vi "Pick Image.vi"(5 "Image to Add [ ]":T1, 9 "String":string, 11 "error in (no error)":errorcluster) -> (4 "InstanceImage":refnum<k24>, 6 "Valid Image?":bool, 8 "String OUT":string, 10 "Change Font Color?":bool, 15 "error out":errorcluster)   [LabVIEW 2012]
doc: "Version 1.0\nDeveloped by Jean-Marc Simard\nCopyright © 2010, Exaprom Inc.\nAll rights reserved.\nLicense: BSD\n\nWith iTextSharp 4.1.6 (http://itextsharp.sourceforge.net)\nunder Mozilla Public License Version 1.1\n(http://www.mozilla.org/MPL/MPL-1.1.html)"
uses:
  Controls/Image to Add refnum [ ].ctl
  C:/Users/MaxCorp/Documents/TopPerm - Base/DLL/itextsharp.dll
  DLL/itextsharp.dll
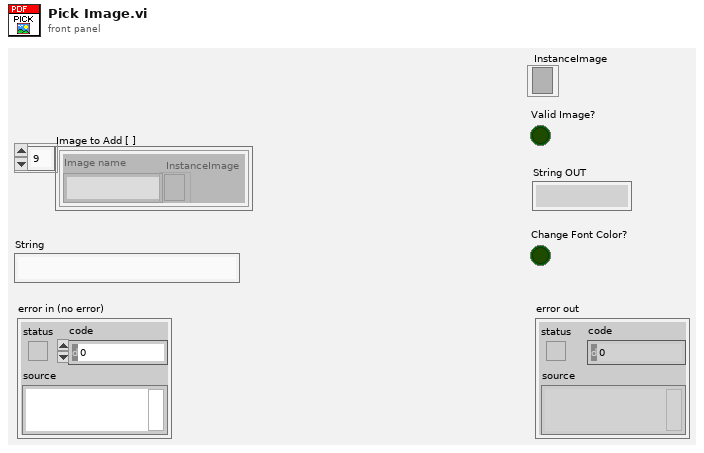
[diagram p1: front panel]
types:
  T1 = typedef "Image to Add refnum [ ].ctl" = cluster{"Image name":string, "InstanceImage":refnum<k24>}[]
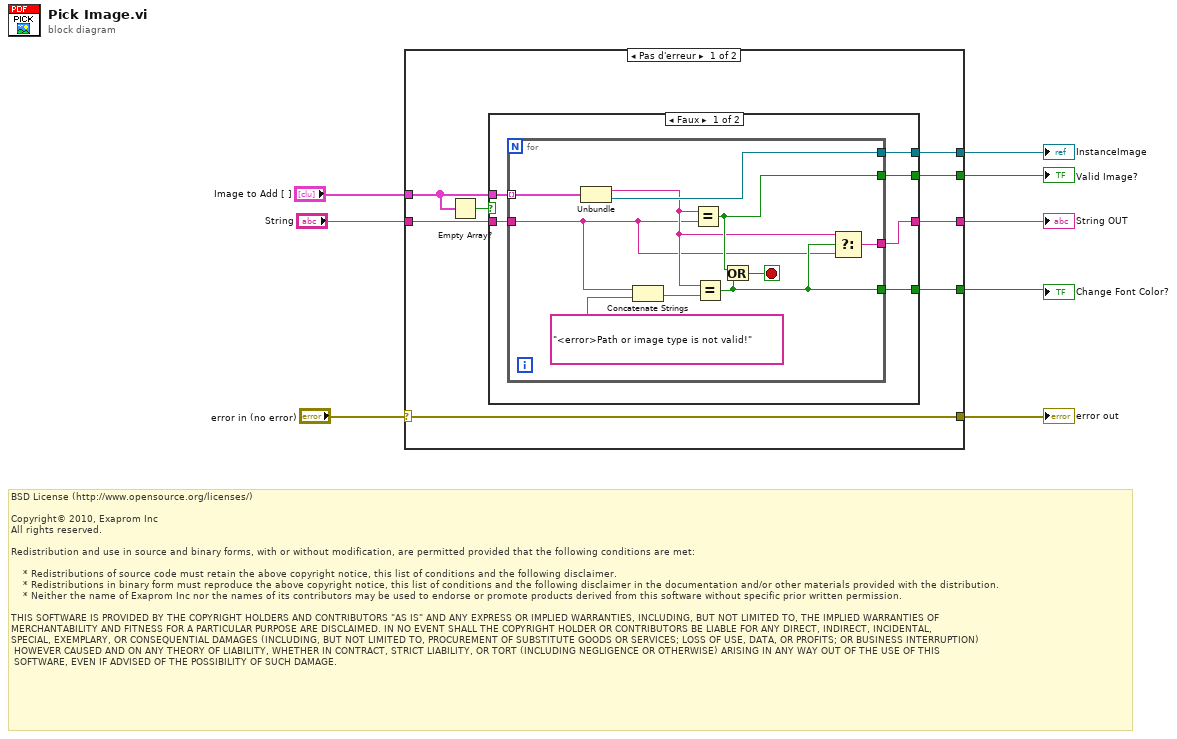
[diagram p0: block diagram]
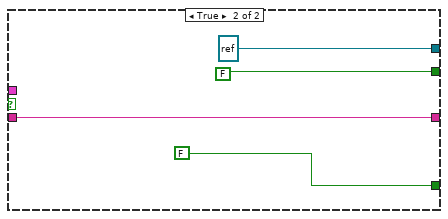
[diagram p2: hidden frame]
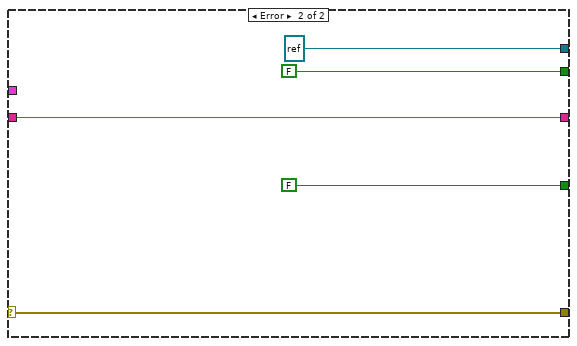
[diagram p3: hidden frame]
diagram:
  # "BSD License (http://www.opensource.org/licenses/)\n\nCopyright© 2010, Exaprom Inc\nAll rights reserved.\n\nRedistribution and use in source and binary forms, with or without modification, are permitted provided that the following conditions are met:\n\n    * Redistributions of source code must retain the above copyright notice, this list of conditions and the following disclaimer.\n    * Redistributions in binary form must reproduce the above copyright notice, this list of conditions and the following disclaimer in the documentation and/or other materials provided with the distribution.\n    * Neither the name of Exaprom Inc nor the names of its contributors may be used to endorse or promote products derived from this software without specific prior written permission.\n\nTHIS SOFTWARE IS PROVIDED BY THE COPYRIGHT HOLDERS AND CONTRIBUTORS \"AS IS\" AND ANY EXPRESS OR IMPLIED WARRANTIES, INCLUDING, BUT NOT LIMITED TO, THE IMPLIED WARRANTIES OF \nMERCHANTABILITY AND FITNESS FOR A PARTICULAR PURPOSE ARE DISCLAIMED. IN NO EVENT SHALL THE COPYRIGHT HOLDER OR CONTRIBUTORS BE LIABLE FOR ANY DIRECT, INDIRECT, INCIDENTAL,\nSPECIAL, EXEMPLARY, OR CONSEQUENTIAL DAMAGES (INCLUDING, BUT NOT LIMITED TO, PROCUREMENT OF SUBSTITUTE GOODS OR SERVICES; LOSS OF USE, DATA, OR PROFITS; OR BUSINESS INTERRUPTION)\n HOWEVER CAUSED AND ON ANY THEORY OF LIABILITY, WHETHER IN CONTRACT, STRICT LIABILITY, OR TORT (INCLUDING NEGLIGENCE OR OTHERWISE) ARISING IN ANY WAY OUT OF THE USE OF THIS\n SOFTWARE, EVEN IF ADVISED OF THE POSSIBILITY OF SUCH DAMAGE."
  n1 = case shown="Pas d'erreur" "error in (no error)" {
    selector: "error in (no error)" -> [w16 w41]
    tunnel: [w16 w41] -> w8
    tunnel: "Image to Add [ ]" -> [w14 _]
    tunnel: "String" -> [w13 w38]
    tunnel: [w12 refnum<k24> refnum ("InstanceImage")] -> w4
    tunnel: [w11 FALSE] -> w3
    tunnel: [w10 w38] -> w2
    tunnel: [w9 FALSE] -> w1
    frame No Error {
      n2 = Empty Array?(array=w14) -> (empty?=w15:bool)
      n3 = case shown="Faux" w15 {
        tunnel: w13 -> [w22 w33]
        tunnel: w14 -> [w21 _]
        tunnel: [w20 refnum<k24> refnum ("InstanceImage")] -> w12
        tunnel: [w19 FALSE] -> w9
        tunnel: [w18 FALSE] -> w11
        tunnel: [w17 w33] -> w10
        frame False {
          n4 = for {
            tunnel: w21 -> [w32] mode=indexing
            tunnel: w22 -> [w23]
            tunnel: [w31] -> w20
            tunnel: [w25] -> w19
            tunnel: [w27] -> w18
            tunnel: [w26] -> w17
            stop <- w28 stop-if-true
            n5 = Unbundle(w32) -> ("Image name"=w24:string, "InstanceImage"=w31:refnum<k24>)
            n6 = Concatenate Strings(w23, "<error>Path or image type is not valid!") -> (w29:string)
            n7 = Equal?(x=w24, y=w23) -> (x = y?=w27:bool)
            n8 = Equal?(x=w24, y=w29) -> (x = y?=w25:bool)
            n9 = Or(x=w27, y=w25) -> (x .or. y?=w28:bool)
            n10 = Select(t=w24, s=w25, f=w23) -> (s? t:f=w26:string)
          }
        }
        frame True {
        }
      }
    }
    frame Error {
    }
  }
  "error out" <- w8
  "InstanceImage" <- w4
  "Valid Image?" <- w3
  "String OUT" <- w2
  "Change Font Color?" <- w1
